vi "qc4_rafik_psm_Aurduino2.vi"() -> ()   [LabVIEW 2020]
uses:
  <instrlib>/CAEN PSM/CAEN PSM.lvlib
panel:
  in  "Voltage Max (0.0 V) 2":u16 max=9999
  in  "Voltage ramp up (0 V/s)":u16 max=999
  in  "Voltage Max (0.0 V)":u16 max=9999
  out "millisecond timer value":u32
  in  "Parameter name":string
  in  "Board parameter? (F)":bool
  out "Parameter descriptor":T1
  out "VMon display":dbl[](array[numeric]) format="%.1f"
  out "Vset DISP":dbl
  out "loop count":i32
  out "IMon values (uA)":dbl[][](array[numeric])
  out "Req (cal Mohm)":dbl[][](array[numeric])
  out "VMon values (V)":dbl[][](array[numeric])
  in  "Enable (OFF)":bool
  in  "Vinital Value(V)":dbl
  in  "Req (Mohm)":dbl
  in  "Board Address":i8
  in  "Channel (0)":u8
  in  "CAEN N1470/1471 PORT":refnum<visa-resource-name>
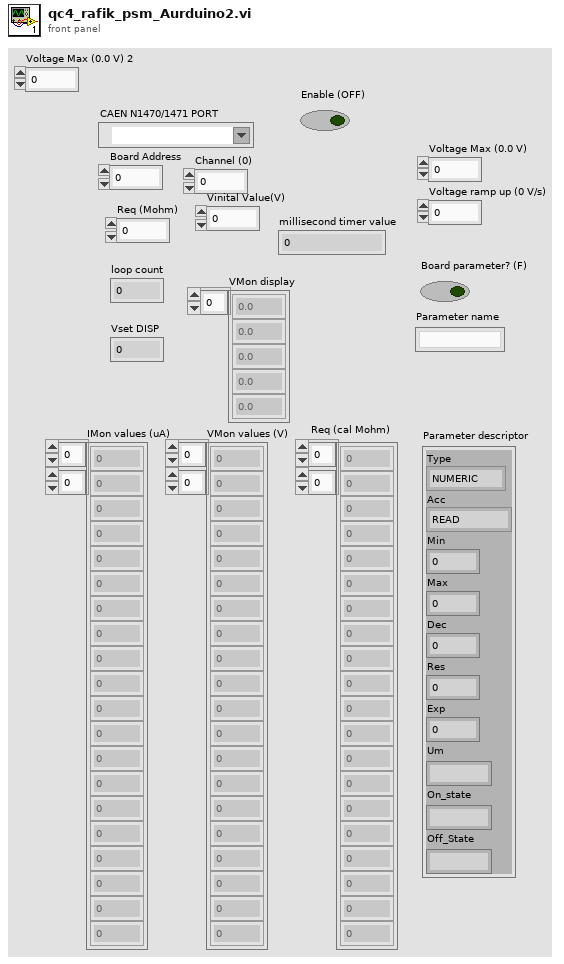
[diagram p1: front panel]
types:
  T1 = cluster{"Type":enum16{"NUMERIC", "ONOFF", "CHSTATUS", "BDSTATUS", "BINARY", "STRING", "ENUM"}, "Acc":enum16{"READ", "WRITE", "READ_WRITE"}, "Min":u32, "Max":u32, "Dec":u32, "Res":u32, "Exp":i32, "Um":string, "On_state":string, "Off_State":string}
  T2 = cluster{"Baud Rate":u32, "Parity":enum16{"None", "Odd", "Even", "Mark", "Space"}, "Data Bits":u16, "Stop Bits":u16, "Flow Control":u16}
  T3 = typedef "CAEN PSM.lvlib/BoardHandle.ctl" = cluster{"VISA resource name":refnum<visa-resource-name>, "Board address":i8, "NChannels":u8}
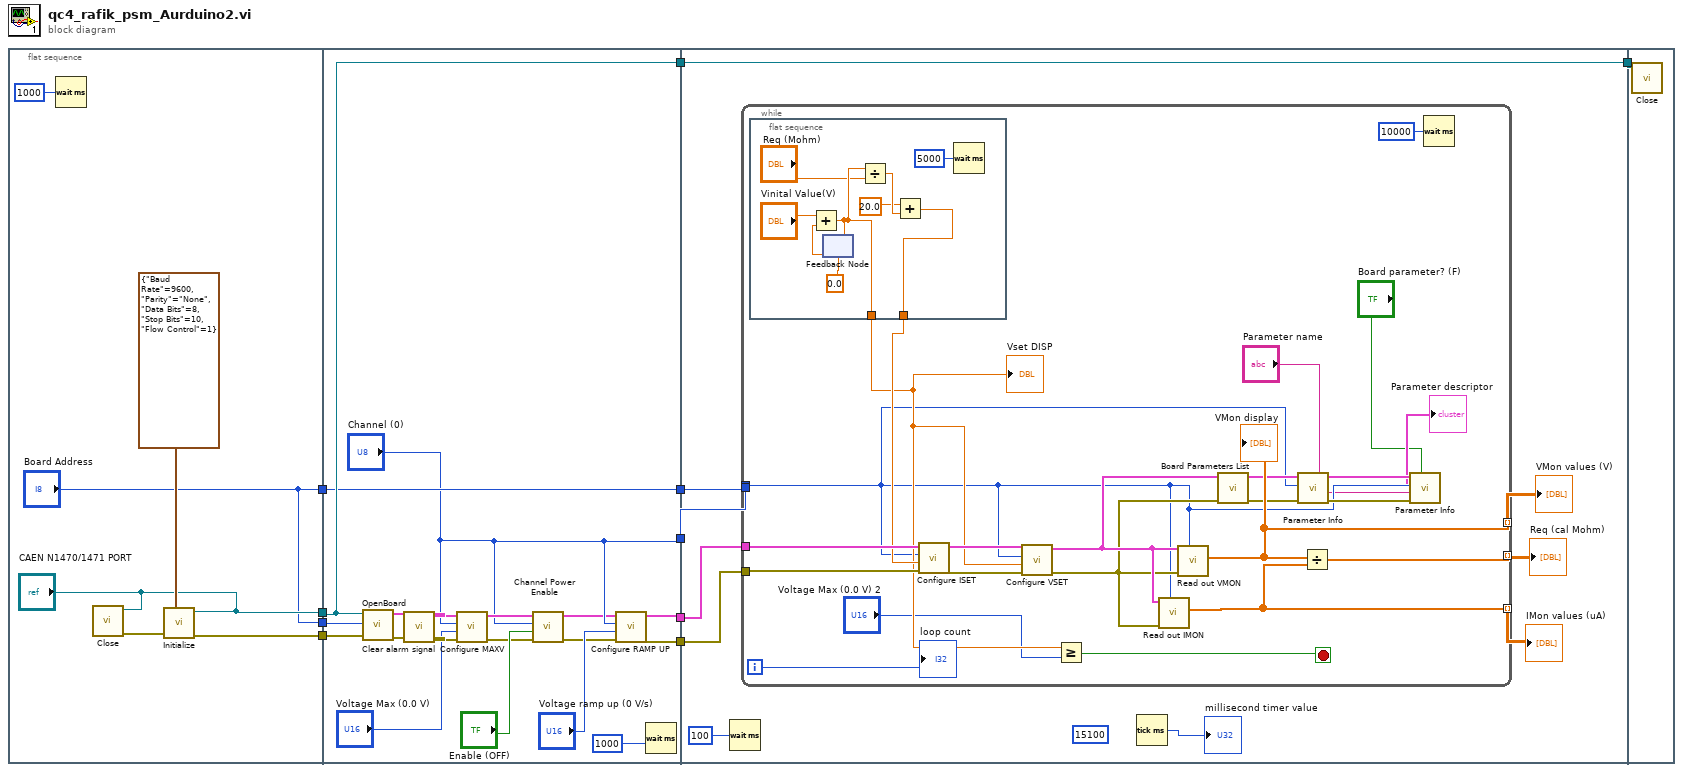
[diagram p0: block diagram]
diagram:
  n1 = flat-sequence {
    tunnel: [w13] -> w10
    tunnel: ["CAEN N1470/1471 PORT"] -> w9
    tunnel: ["Board Address"] -> w7
    tunnel: ["Board Address"] -> w5
    tunnel: w10 -> [w35]
    tunnel: w9 -> [w34]
    tunnel: [w34] -> w8
    tunnel: w7 -> [w33]
    tunnel: [w33] -> w6
    tunnel: w5 -> [w30]
    tunnel: [w18] -> w4
    tunnel: ["Channel (0)"] -> w3
    tunnel: [w17] -> w1
    tunnel: w8 -> [w40]
    tunnel: w6 -> [w38]
    tunnel: w4 -> [w43]
    tunnel: w3 -> [w45]
    tunnel: [w40] -> w2
    tunnel: w1 -> [w44]
    tunnel: w2 -> [w78]
    frame #0 {
      n2 = Wait (ms)(milliseconds to wait=u32 1000) -> ()  [unwired: 1 out]
      n3 = call <instrlib>:"Close.vi"("VISA resource name"="CAEN N1470/1471 PORT") -> ("error out"=w16:errorcluster)  [unwired: 10 in]
      n4 = call <instrlib>:"Initialize.vi"("Serial Configuration"=T2 {"Baud Rate"=9600, "Parity"=enum."None", "Data Bits"=8, "Stop Bits"=10, "Flow Control"=1}, "error in (no error)"=w16, "VISA resource name"="CAEN N1470/1471 PORT") -> ("error out"=w13:errorcluster)  [unwired: 7 in, 1 out]
    }
    frame #1 {
      n5 = call <instrlib>:"OpenBoard.vi"("error in (no error)"=w35, "Board Address"=w30, "VISA resource name"=w34) -> ("error out"=w31:errorcluster, "BoardHandle"=w32:T3)  [unwired: 7 in]
      n6 = call <instrlib>:"Clear alarm signal.vi"("error in (no error)"=w31, "BoardHandle"=w32) -> ("error out"=w25:errorcluster, "BoardHandle out"=w27:T3)  [unwired: 8 in]
      n7 = call <instrlib>:"Configure MAXV.vi"("error in (no error)"=w25, "Voltage Max (0.0 V)"="Voltage Max (0.0 V)", "Channel (0)"="Channel (0)", "BoardHandle"=w27) -> ("error out"=w24:errorcluster, "BoardHandle out"=w26:T3)  [unwired: 6 in]
      n8 = call <instrlib>:"Channel Power Enable.vi"("error in (no error)"=w24, "Enable (OFF)"="Enable (OFF)", "Channel (0)"="Channel (0)", "BoardHandle"=w26) -> ("error out"=w19:errorcluster, "BoardHandle out"=w20:T3)  [unwired: 6 in]
      n9 = call <instrlib>:"Configure RAMP UP.vi"("error in (no error)"=w19, "Voltage ramp up (0 V/s)"="Voltage ramp up (0 V/s)", "Channel (0)"="Channel (0)", "BoardHandle"=w20) -> ("error out"=w17:errorcluster, "BoardHandle out"=w18:T3)  [unwired: 6 in]
      n10 = Wait (ms)(milliseconds to wait=u32 1000) -> ()  [unwired: 1 out]
    }
    frame #2 {
      (unwired) u32 15100 ("millisecond timer value")
      n11 = Wait (ms)(milliseconds to wait=u32 100) -> ()  [unwired: 1 out]
      n12 = while {
        tunnel: w45 -> [w50]
        tunnel: w44 -> [w65]
        tunnel: w43 -> [w64]
        tunnel: [w62] -> w42 mode=indexing
        tunnel: [w61] -> w39 mode=indexing
        tunnel: [w60] -> w41 mode=indexing
        tunnel: w38 -> [_]
        i -> [w57]
        stop <- w58 stop-if-true
        n13 = flat-sequence {
          tunnel: [w77] -> w63
          tunnel: [w76] -> w59
          frame #0 {
            n14 = feedback #1(0.0) -> (w74:dbl)
            n15 = Add(x="Vinital Value(V)", y=w74) -> (x+y=w76:dbl)
            n16 = feedback-in #1(w76) -> ()
            n17 = Divide(x=w76, y="Req (Mohm)") -> (x/y=w72:dbl)
            n18 = Add(x=20.0, y=w72) -> (x+y=w77:dbl)
            n19 = Wait (ms)(milliseconds to wait=u32 5000) -> ()  [unwired: 1 out]
          }
        }
        n20 = call <instrlib>:"Configure ISET.vi"("error in (no error)"=w65, "Current Limit (0.00 uA)"=w63, "Channel (0)"=w50, "BoardHandle"=w64) -> ("error out"=w67:errorcluster, "BoardHandle out"=w66:T3)  [unwired: 6 in]
        n21 = call <instrlib>:"Configure VSET.vi"("error in (no error)"=w67, "Voltage Level (0.0 V)"=w59, "Channel (0)"=w50, "BoardHandle"=w66) -> ("error out"=w55:errorcluster, "BoardHandle out"=w68:T3)  [unwired: 6 in]
        n22 = Greater Or Equal?(x=w59, y="Voltage Max (0.0 V) 2") -> (x >= y?=w58:bool)
        n23 = call <instrlib>:"Read out IMON.vi"("Channel"=w50, "error in (no error)"=w55, "BoardHandle"=w68) -> ("IMon values (uA)"=w60:dbl[])  [unwired: 5 in, 3 out]
        n24 = call <instrlib>:"Read out VMON.vi"("Channel"=w50, "error in (no error)"=w55, "BoardHandle"=w68) -> ("VMon values (V)"=w61:dbl[])  [unwired: 6 in, 2 out]
        "VMon display" <- w61
        n25 = call <instrlib>:"Board Parameters List.vi"("error in (no error)"=w55, "BoardHandle"=w68) -> ("error out"=w53:errorcluster, "BoardHandle out"=w54:T3)  [unwired: 6 in, 2 out]
        n26 = call <instrlib>:"Parameter Info.vi"("error in (no error)"=w53, "Parameter name"="Parameter name", "Channel"=w50, "BoardHandle"=w54) -> ("error out"=w51:errorcluster, "BoardHandle out"=w52:T3)  [unwired: 5 in, 1 out]
        n27 = Divide(x=w61, y=w60) -> (x/y=w62:dbl[])
        n28 = call <instrlib>:"Parameter Info.vi"("Board parameter? (F)"="Board parameter? (F)", "error in (no error)"=w51, "Parameter name"="Parameter name", "Channel"=w50, "BoardHandle"=w52) -> ("Parameter descriptor"=→"Parameter descriptor":T1)  [unwired: 4 in, 2 out]
        n29 = Wait (ms)(milliseconds to wait=u32 10000) -> ()  [unwired: 1 out]
        "loop count" <- w57
        "Vset DISP" <- w59
      }
      "VMon values (V)" <- w39
      "Req (cal Mohm)" <- w42
      "IMon values (uA)" <- w41
      n30 = Tick Count (ms)() -> (millisecond timer value=→"millisecond timer value":u32)
    }
    frame #3 {
      n31 = call <instrlib>:"Close.vi"("VISA resource name"=w78) -> ()  [unwired: 10 in, 1 out]
    }
  }
